vi "Check Movement Against Limits.vi"(6 "Height of Menu Pane":i32, 8 "error in":errorcluster, 9 "Maximum Distance Away From Sides":i32, 10 "Distance Mouse Moved":i32, 11 "Display State In":T1 caption="State") -> (0 "error out":errorcluster, 2 "Distance to Move":i32, 3 "Display State In Out":T1={"Numeric"=0.0, "Array of Button References"=[], "Space Between Menu Buttons"=3, "Number of Menu Buttons"=6, "Array of Button Names"=[], "Most Recent Vertical Position"=0, "This VI"=refnum, "Current Action"=enum."Not Moving", "Most Recent Distance Traveled"=0, "Method"=enum."Resize", "Data In"=0} caption="State")   [LabVIEW 2011, in "Sliding Menu Library.lvlib" / "Sliding Menu XControl.xctl"]
uses:
  Sliding Menu XControl.xctl
  Sliding Menu State.ctl
  Menu Button Library/Menu Button xControl/Menu Button xControl.xctl
  Sliding Menu SubVIs/Sliding Menu Type Definitions/Current User Action.ctl
  Sliding Menu Methods.ctl
  Sliding Menu Data.ctl
  Sliding Menu Library.lvlib
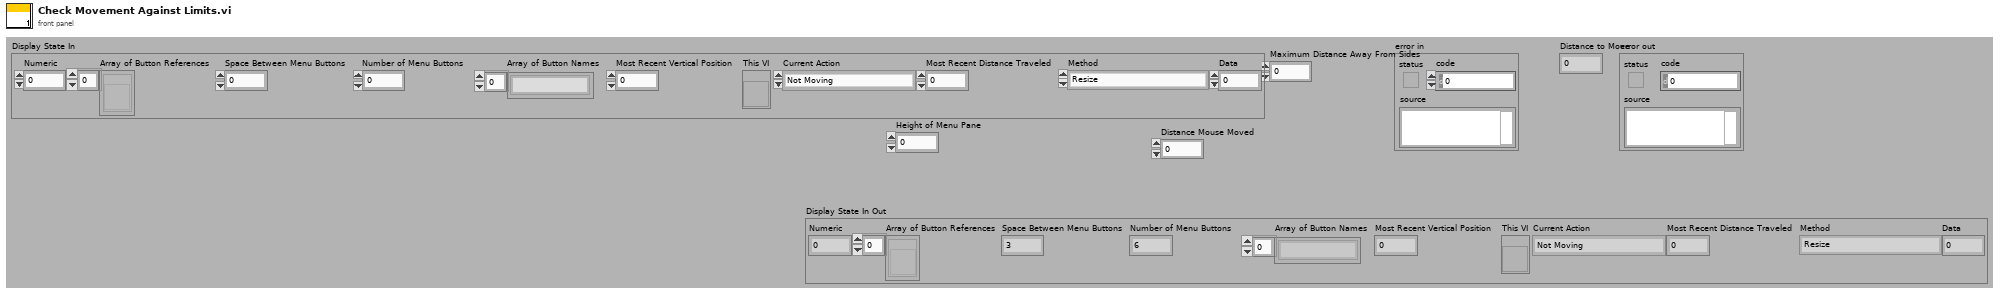
[diagram p1: front panel]
types:
  T1 = typedef "Sliding Menu Library.lvlib/Sliding Menu XControl.xctl/Sliding Menu State.ctl" = cluster{"Numeric":dbl, "Array of Button References":refnum<vi>[], "Space Between Menu Buttons":i32, "Number of Menu Buttons":i32, "Array of Button Names":string[], "Most Recent Vertical Position":i32, "This VI":refnum<vi>, "Current Action":T2, "Most Recent Distance Traveled":i32, "Method":T3, "Data In":T4}
  T2 = typedef "Sliding Menu Library.lvlib/Current User Action.ctl" = enum16{"Not Moving", "Mouse Down", "Mouse Up No Dragging", "Bounce Up Needed", "Bounce Down Needed", "Dragging", "Easing"}
  T3 = typedef "Sliding Menu Methods.ctl" = enum16{"Resize", "Move Up", "Move Down", "Move to 0"}
  T4 = typedef "Sliding Menu Library.lvlib/Sliding Menu XControl.xctl/Sliding Menu Data.ctl" = i32
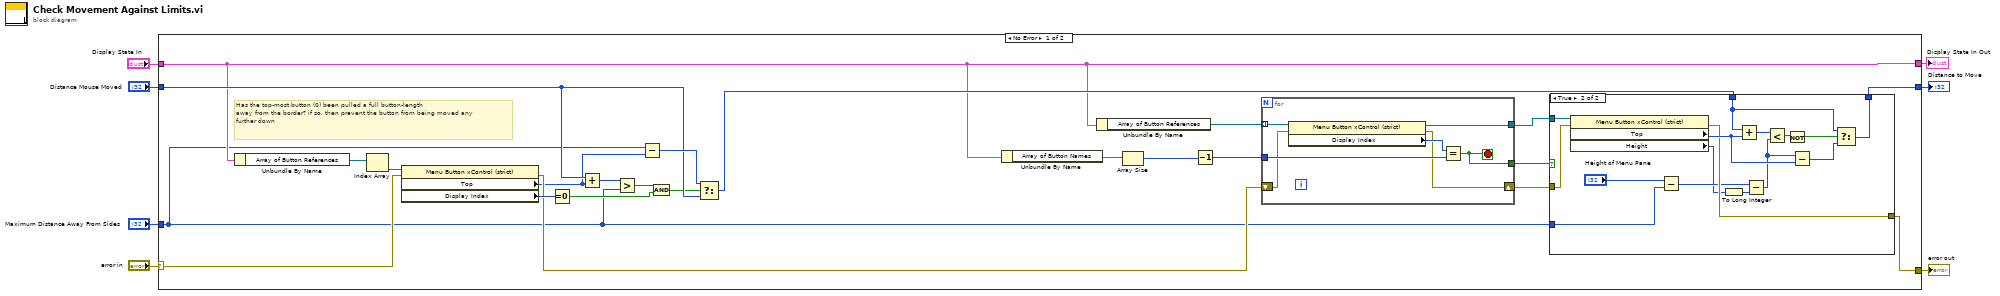
[diagram p0: block diagram]
diagram:
  n1 = case shown="No Error" "error in" {
    selector: "error in" -> [w23 _]
    tunnel: [w13 _] -> w7
    tunnel: "Maximum Distance Away From Sides" -> [w8 _]
    tunnel: [w14 _] -> w5
    tunnel: "Distance Mouse Moved" -> [w30 _]
    tunnel: "Display State In" -> [w11 _]
    tunnel: [w11 _] -> w1
    frame No Error {
      # "Has the top-most button (0) been pulled a full button-length\naway from the border? if so, then prevent the button from being moved any further down"
      n2 = Unbundle By Name(w11) -> ("Array of Button References"=w24:refnum<vi>[])
      n3 = Index Array(array=w24) -> (element=w25:refnum<vi>)  [unwired: 1 in]
      n4 = property class="Menu Button xControl (strict)"(reference=w25, error in=w23) -> (error out=w18:errorcluster, "Top"=w9:i32, "Display Index"=w26:i32)  [unwired: 1 out]
      n5 = Equal To 0?(x=w26) -> (x = 0?=w29:bool)
      n6 = Add(x=w30, y=w9) -> (x+y=w27:i32)
      n7 = Greater?(x=w27, y=w8) -> (0:w28:bool)
      n8 = Subtract(x=w8, y=w9) -> (x-y=w31:i32)
      n9 = And(x=w28, y=w29) -> (x .and. y?=w10:bool)
      n10 = Select(t=w31, s=w10, f=w30) -> (s? t:f=w12:i32)
      n11 = Unbundle By Name(w11) -> ("Array of Button Names"=w22:string[])
      n12 = Unbundle By Name(w11) -> ("Array of Button References"=w21:refnum<vi>[])
      n13 = Array Size(array=w22) -> (size(s)=w20:i32)
      n14 = Decrement(x=w20) -> (x-1=w19:i32)
      n15 = for {
        tunnel: w21 -> [w56] mode=indexing
        tunnel: w19 -> [w54]
        tunnel: [w53] -> w16
        shift-right: [w52] -> w15
        shift-left: w18 -> [w51]
        tunnel: [w50] -> w17
        stop <- w50 stop-if-true
        n16 = property class="Menu Button xControl (strict)"(reference=w56, error in=w51) -> (reference out=w53:refnum<vi>, error out=w52:errorcluster, "Display Index"=w55:i32)
        n17 = Equal?(x=w55, y=w54) -> (x = y?=w50:bool)
      }
      n18 = case shown="True" w17 {
        tunnel: w16 -> [_ w49]
        tunnel: w15 -> [w32 w41]
        tunnel: w12 -> [w33 w45]
        tunnel: [w33 w47] -> w14
        tunnel: [w32 w40] -> w13
        tunnel: w8 -> [_ w38]
        frame False {
        }
        frame True {
          n19 = property class="Menu Button xControl (strict)"(reference=w49, error in=w41) -> (error out=w40:errorcluster, "Top"=w43:i32, "Height"=w35:u32)  [unwired: 1 out]
          n20 = Subtract(x="Height of Menu Pane", y=w38) -> (x-y=w37:i32)
          n21 = To Long Integer(number=w35) -> (32bit integer=w34:i32)
          n22 = Add(x=w45, y=w43) -> (x+y=w48:i32)
          n23 = Subtract(x=w37, y=w34) -> (x-y=w36:i32)
          n24 = Less?(x=w48, y=w36) -> (x < y?=w46:bool)
          n25 = Not(x=w46) -> (.not. x?=w44:bool)
          n26 = Subtract(x=w36, y=w43) -> (x-y=w42:i32)
          n27 = Select(t=w45, s=w44, f=w42) -> (s? t:f=w47:i32)
        }
      }
    }
    frame Error {
    }
  }
  "error out" <- w7
  "Distance to Move" <- w5
  "Display State In Out" <- w1
